vi "DAC Init Results.vi"(8 "error in":errorcluster, 9 "Log Details?":bool, 10 "tdms file":refnum<k34>, 11 "DAC Heater Box Temperatures in":refnum<class "DAC Pressure Scan.lvclass">) -> (0 "error out":errorcluster, 2 "tdms file out":refnum<k34>)   [LabVIEW 2019, in "DAC.lvlib" / "DAC Pressure Scan.lvclass"]
uses:
  DAC Pressure Scan.lvclass
  C:/Users/krio/Documents/LV_Projects/test-stand/App/DAC/DAC.lvclass
  DAC.lvclass/DAC.ctl
  DAC Pressure Scan.lvclass/DAC Pressure Scan.ctl
  DAC.lvclass
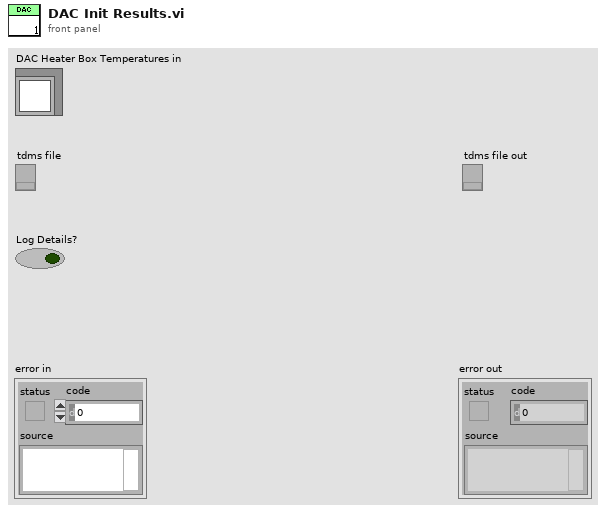
[diagram p1: front panel]
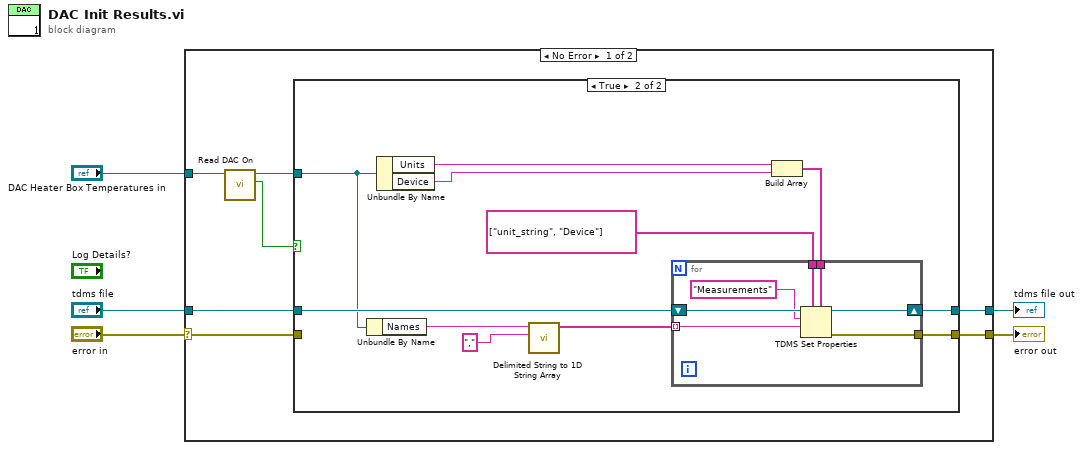
[diagram p0: block diagram]
diagram:
  n1 = case shown="No Error" "error in" {
    selector: "error in" -> [w6 w34]
    tunnel: [w10 w34] -> w2
    tunnel: "DAC Heater Box Temperatures in" -> [w9 _]
    tunnel: "tdms file" -> [w12 w33]
    tunnel: [w11 w33] -> w1
    frame No Error {
      n2 = call "Read DAC On.vi"("DAC in"=w9) -> ("DAC On"=w7:bool, "DAC in"=w8:refnum<class "DAC Pressure Scan.lvclass">)  [unwired: 8 in, 1 out]
      n3 = case shown="True" w7 {
        tunnel: w12 -> [w14 w25]
        tunnel: [w14 w23] -> w11
        tunnel: [w13 w22] -> w10
        tunnel: w8 -> [_ w19]
        tunnel: w6 -> [w13 _]
        frame False {
        }
        frame True {
          n4 = Unbundle By Name(w19) -> ("Names"=w18:string)
          n5 = Unbundle By Name(w19) -> ("Units"=w17:string, "Device"=w15:string)
          n6 = call <vilib>:"Delimited String to 1D String Array.vi"("delimiter"=",", "delimited string"=w18) -> ("string array"=w21:string[])  [unwired: 9 in]
          n7 = Build Array(w17, w15) -> (w16:string[])
          n8 = for {
            tunnel: w21 -> [w30] mode=indexing
            tunnel: string[] ["unit_string", "Device"] ("property names") -> [w29]
            tunnel: w16 -> [w28]
            tunnel: [w26] -> w22
            shift-right: [w27] -> w23
            shift-left: w25 -> [w32]
            n9 = TDMS Set Properties(5:w28, 7:w29, 9:w30, 10:"Measurements" ("group name in (Untitled)"), 11:w32) -> (0:w26:errorcluster, 3:w27:refnum<k34>)  [unwired: 1 in, 2 out]
          }
        }
      }
    }
    frame Error {
    }
  }
  "error out" <- w2
  "tdms file out" <- w1
